vi "Drive Angle_Straight.vi"(1 "Z axis in":dbl, 2 "XAxisIn":dbl, 3 "y input":dbl) -> (8 "Z out":dbl, 9 "X0AxisOut":dbl format="%.2f", 10 "y Output":dbl)   [LabVIEW 2016]
uses:
  Robot Global Data.vi
  <vilib>/addons/control/pid/pid.llb/PID (DBL).vi
  <vilib>/addons/control/pid/pid.llb/PID Control Input Filter (DBL).vi
  <vilib>/addons/control/pid/NI_PID_pid.lvlib
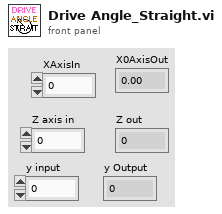
[diagram p1: front panel]
types:
  T1 = typedef "WPI_DriverStationRobotMode2.ctl" = enum16{"Autonomous Disabled", "Autonomous Enabled", "Teleop Disabled", "Teleop Enabled", "Disconnected", "Finish", "Test Disabled", "Test Enabled", "Emergency Stopped"}
  T2 = cluster{"proportional gain (Kc)":dbl, "integral time (Ti, min)":dbl, "derivative time (Td, min)":dbl}
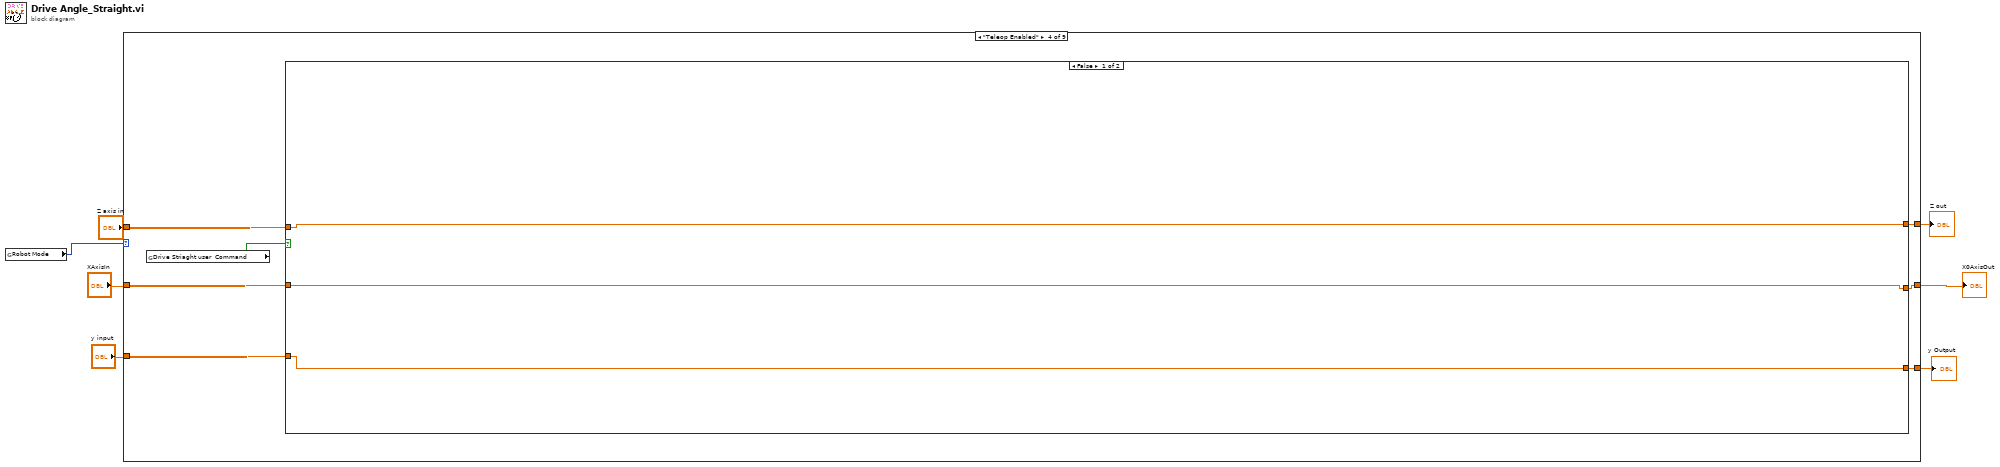
[diagram p0: block diagram]
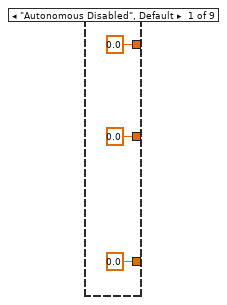
[diagram p2: hidden frame]
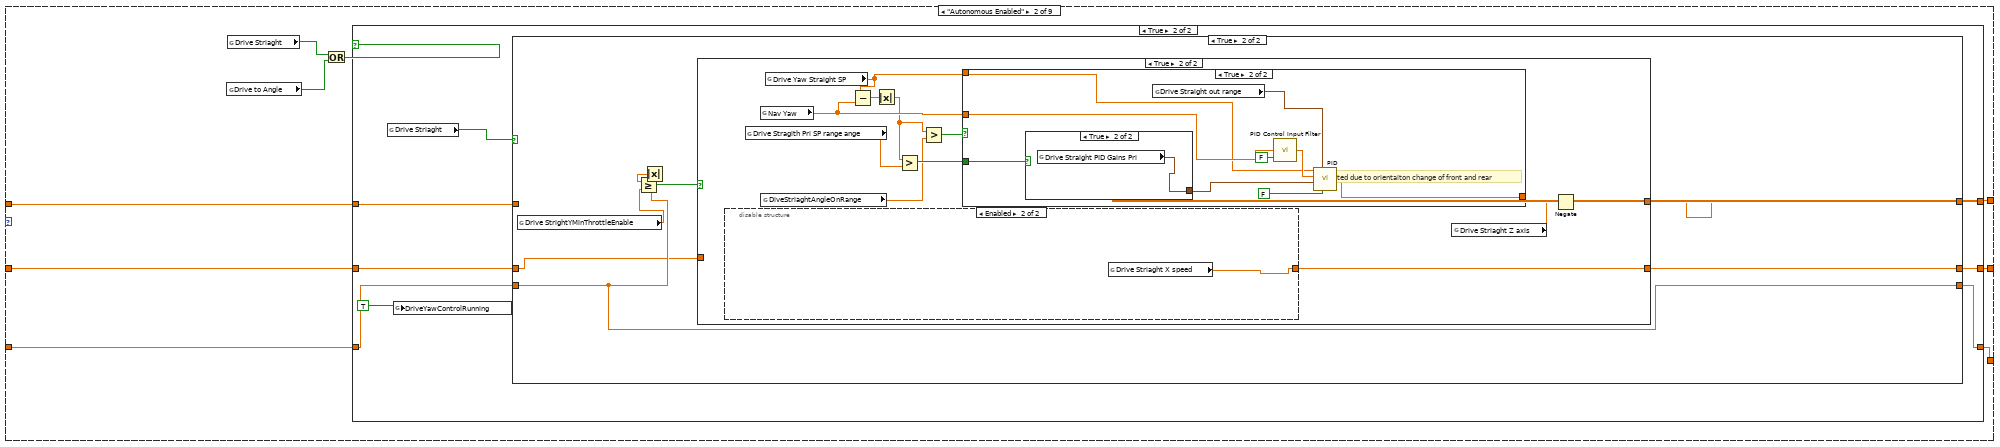
[diagram p3: hidden frame]
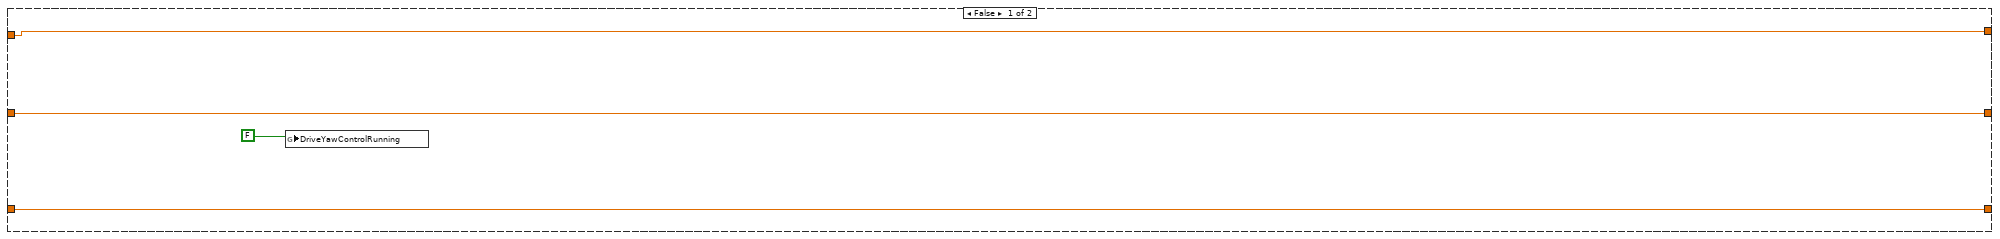
[diagram p4: hidden frame]
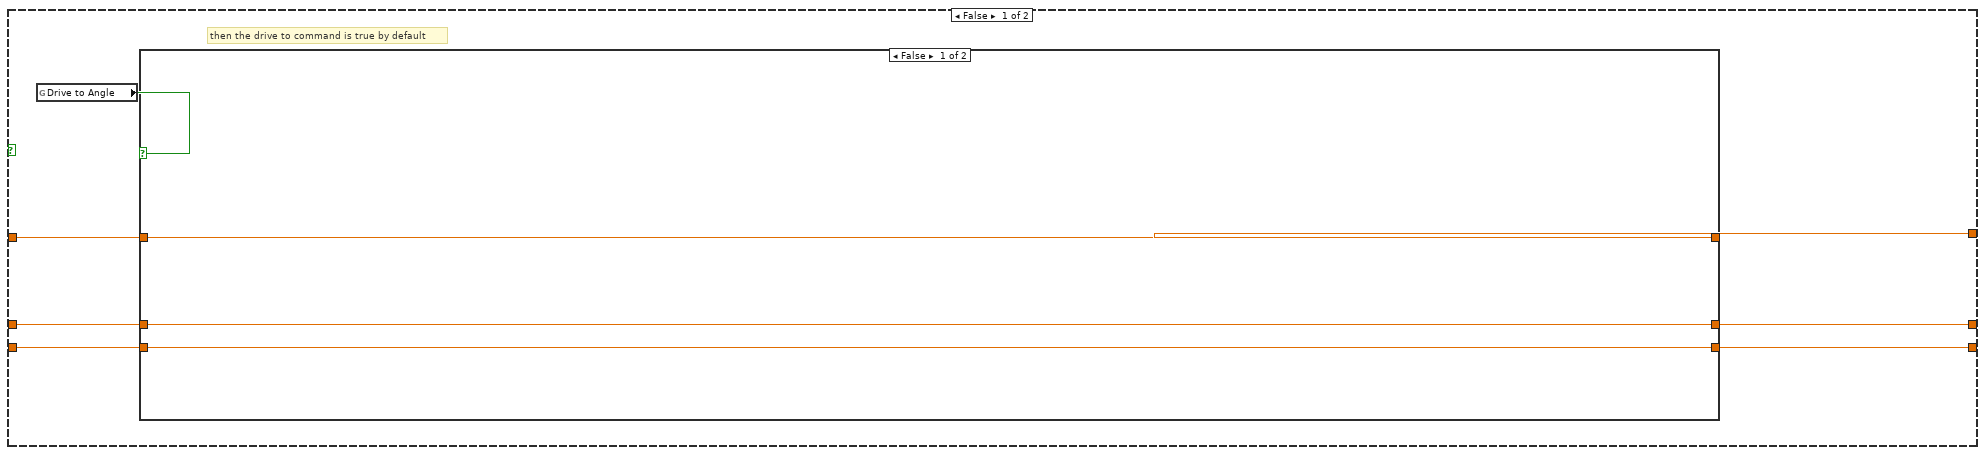
[diagram p5: hidden frame]
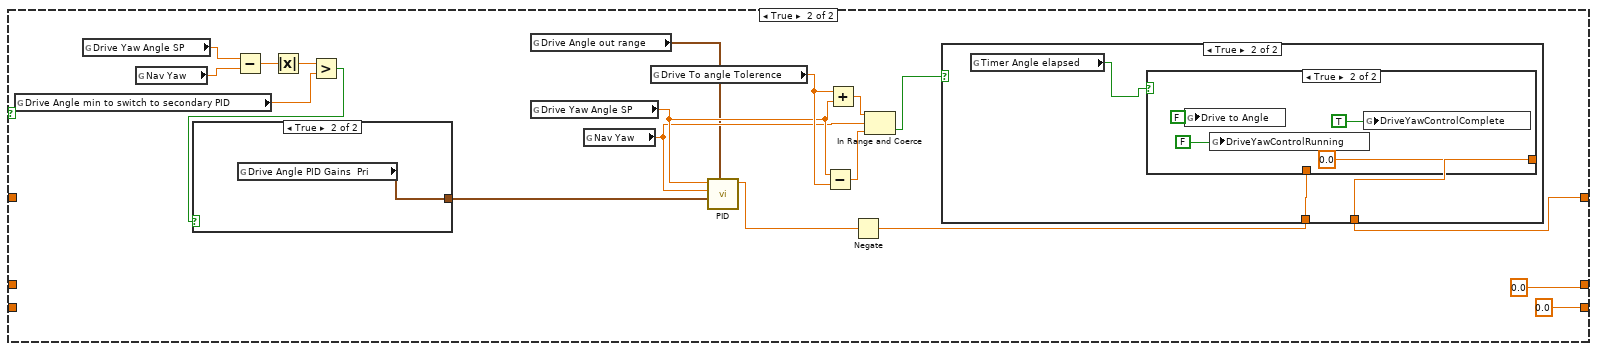
[diagram p6: hidden frame]
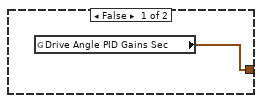
[diagram p7: hidden frame]
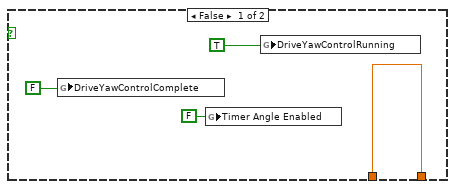
[diagram p8: hidden frame]
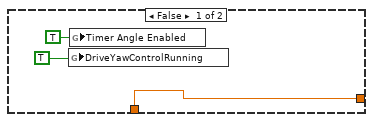
[diagram p9: hidden frame]
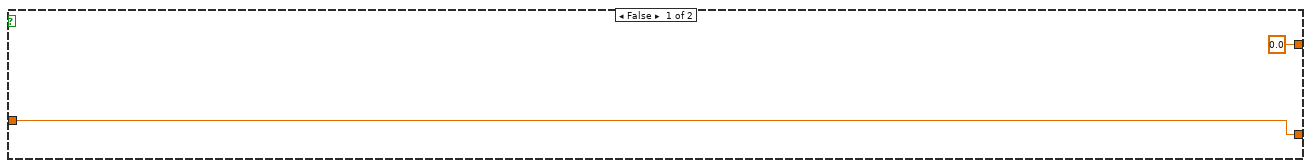
[diagram p10: hidden frame]
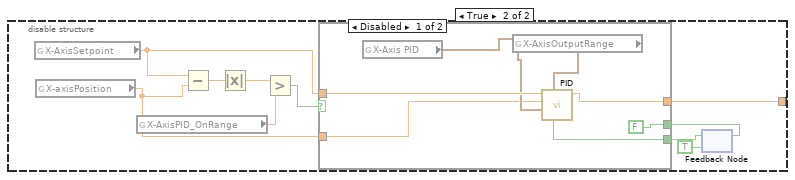
[diagram p11: hidden frame]
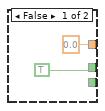
[diagram p12: hidden frame]
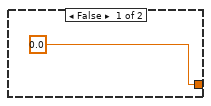
[diagram p13: hidden frame]
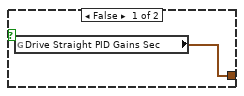
[diagram p14: hidden frame]
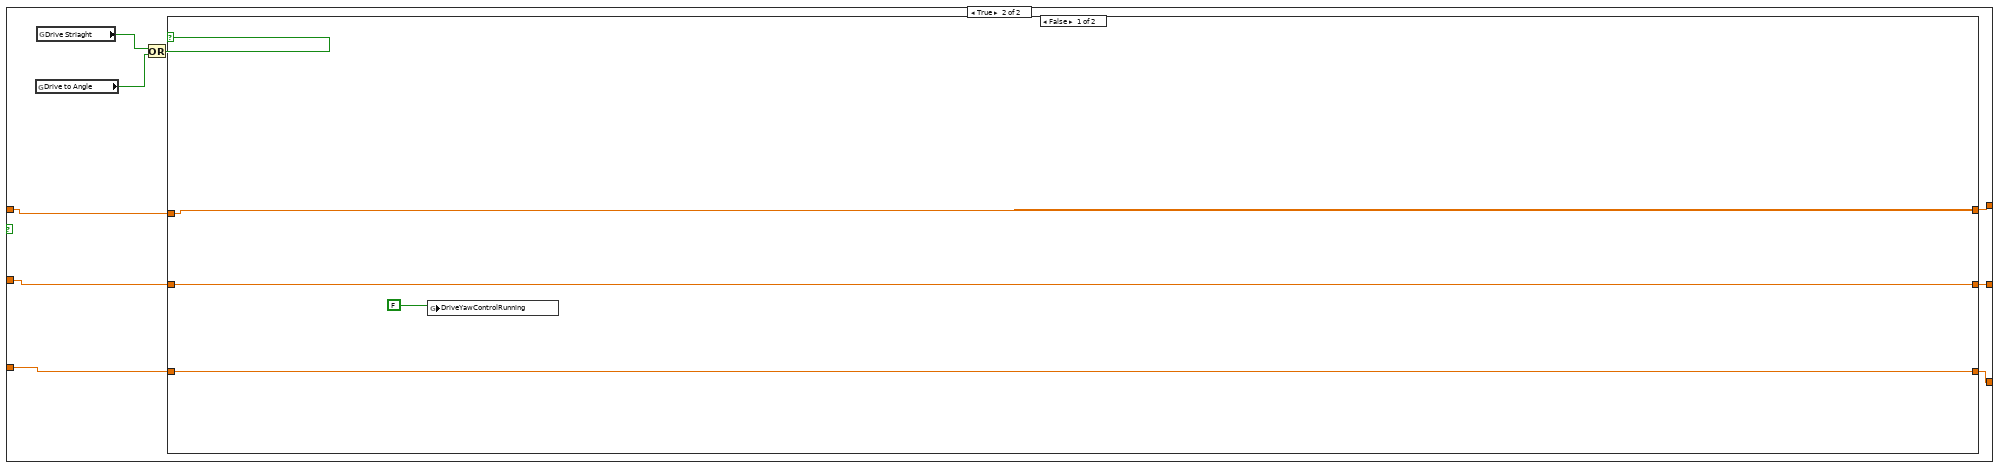
[diagram p16: hidden frame]
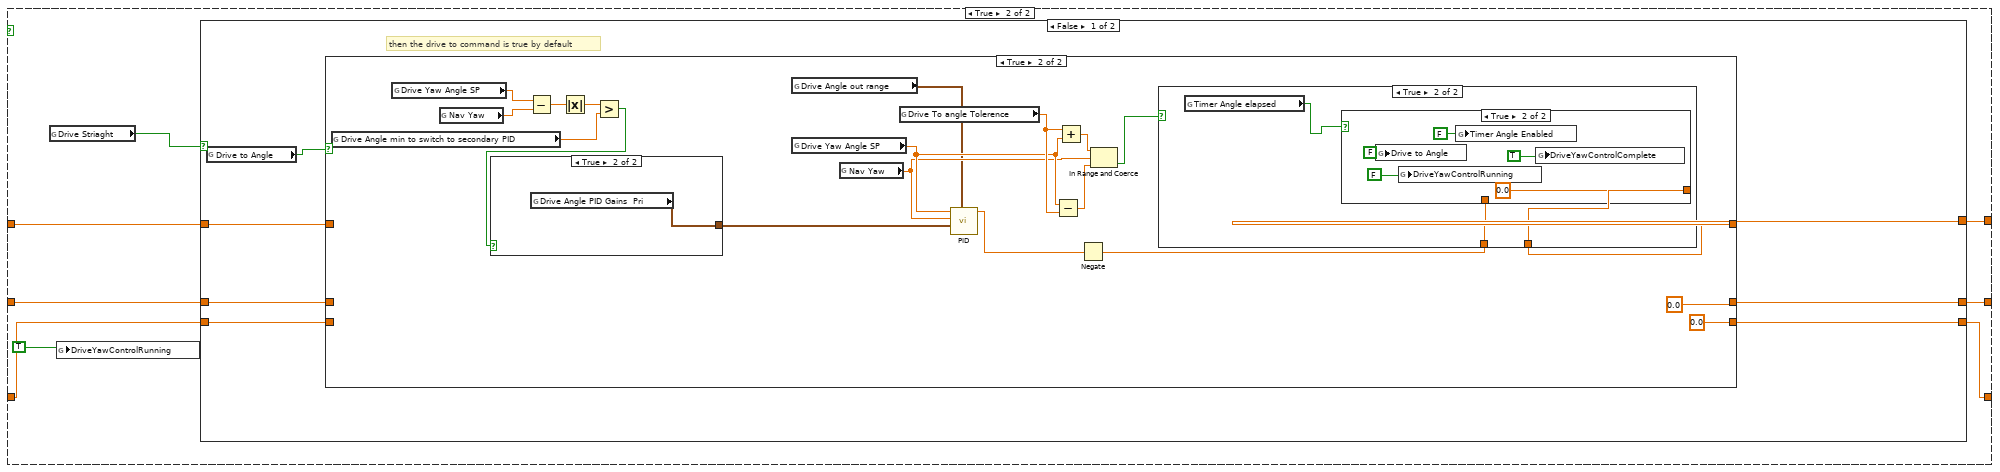
[diagram p17: hidden frame]
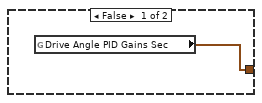
[diagram p19: hidden frame]
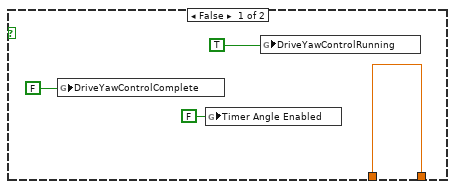
[diagram p20: hidden frame]
diagram:
  n1 = global read "Robot Global Data.vi" "Robot Mode"() -> (w1:T1)
  n2 = case shown="\"Teleop Enabled\"" w1 {
    tunnel: "Z axis in" -> [_ w19 _ w130 _ _ _ _ _]
    tunnel: [0.0 ("Z axis in") w18 _ w135 _ _ _ _ _] -> w6
    tunnel: [0.0 ("Drive Striaght X speed") w14 _ w134 _ _ _ _ _] -> w5
    tunnel: "XAxisIn" -> [_ w13 _ w131 _ _ _ _ _]
    tunnel: "y input" -> [_ w12 _ w132 _ _ _ _ _]
    tunnel: [0.0 ("y input") w11 _ w133 _ _ _ _ _] -> w2
    frame "Autonomous Disabled", Default {
    }
    frame "Autonomous Enabled" {
      n3 = global read "Robot Global Data.vi" "Drive to Angle"() -> (w17:bool)
      n4 = global read "Robot Global Data.vi" "Drive Striaght"() -> (w16:bool)
      n5 = Or(x=w16, y=w17) -> (x .or. y?=w15:bool)
      n6 = case shown="True" w15 {
        tunnel: w19 -> [w23 w29]
        tunnel: [w23 w31] -> w18
        tunnel: [w21 w27] -> w14
        tunnel: w13 -> [w21 w25]
        tunnel: [w20 w26] -> w11
        tunnel: w12 -> [w20 w24]
        frame False {
          n7 = global write "Robot Global Data.vi" "DriveYawControlRunning"(FALSE ("DriveYawControlRunning")) -> ()
        }
        frame True {
          n8 = global read "Robot Global Data.vi" "Drive Striaght"() -> (w30:bool)
          n9 = global write "Robot Global Data.vi" "DriveYawControlRunning"(TRUE ("DriveYawControlRunning")) -> ()
          n10 = case shown="True" w30 {
            tunnel: [w36 w83] -> w31
            tunnel: w29 -> [w37 _]
            tunnel: [w35 w82] -> w27
            tunnel: [w34 w80] -> w26
            tunnel: w25 -> [w33 w77]
            tunnel: w24 -> [w32 w80]
            frame False {
              # "then the drive to command is true by default"
              n11 = global read "Robot Global Data.vi" "Drive to Angle"() -> (w38:bool)
              n12 = case shown="False" w38 {
                tunnel: [w41 w54] -> w36
                tunnel: w37 -> [w41 _]
                tunnel: [w40 0.0 ("output")] -> w35
                tunnel: [w39 0.0 ("output")] -> w34
                tunnel: w33 -> [w40 _]
                tunnel: w32 -> [w39 _]
                frame False {
                }
                frame True {
                  n13 = global read "Robot Global Data.vi" "Drive Angle min to switch to secondary PID"() -> (w46:dbl)
                  n14 = global read "Robot Global Data.vi" "Drive Yaw Angle SP"() -> (w51:dbl)
                  n15 = global read "Robot Global Data.vi" "Nav Yaw"() -> (w50:dbl)
                  n16 = Subtract(x=w51, y=w50) -> (x-y=w49:dbl)
                  n17 = Absolute Value(x=w49) -> (abs(x)=w48:dbl)
                  n18 = Greater?(x=w48, y=w46) -> (0:w47:bool)
                  n19 = case shown="True" w47 {
                    tunnel: [w61 w62] -> w45
                    frame False {
                      n20 = global read "Robot Global Data.vi" "Drive Angle PID Gains Sec"() -> (w61:T2)
                    }
                    frame True {
                      n21 = global read "Robot Global Data.vi" "Drive Angle PID Gains  Pri"() -> (w62:T2)
                    }
                  }
                  n22 = global read "Robot Global Data.vi" "Drive Angle out range"() -> (w52:cluster{"output high":dbl, "output low":dbl})
                  n23 = global read "Robot Global Data.vi" "Drive Yaw Angle SP"() -> (w56:dbl)
                  n24 = global read "Robot Global Data.vi" "Nav Yaw"() -> (w53:dbl)
                  n25 = global read "Robot Global Data.vi" "Drive To angle Tolerence"() -> (w57:dbl)
                  n26 = call-poly <vilib>:"PID.vi"("output range"=w52, "PID gains"=w45, "process variable"=w53, "setpoint"=w56) -> ("output"=w60:dbl)  [unwired: 6 in, 1 out]
                  n27 = Subtract(x=w56, y=w57) -> (x-y=w58:dbl)
                  n28 = Add(x=w57, y=w56) -> (x+y=w59:dbl)
                  n29 = Negate(x=w60) -> (-x=w44:dbl)
                  n30 = In Range and Coerce(upper limit=w59, x=w53, lower limit=w58) -> (In Range?=w55:bool)  [unwired: 1 out]
                  n31 = case shown="True" w55 {
                    tunnel: w44 -> [w65 w68]
                    tunnel: [w65 w69] -> w54
                    frame False {
                      n32 = global write "Robot Global Data.vi" "DriveYawControlComplete"(FALSE ("DriveYawControlRunning")) -> ()
                      n33 = global write "Robot Global Data.vi" "Timer Angle Enabled"(FALSE ("Timer Angle Enabled")) -> ()
                      n34 = global write "Robot Global Data.vi" "DriveYawControlRunning"(TRUE ("DriveYawControlRunning")) -> ()
                    }
                    frame True {
                      n35 = global read "Robot Global Data.vi" "Timer Angle elapsed"() -> (w67:bool)
                      n36 = case shown="True" w67 {
                        tunnel: [w72 0.0] -> w69
                        tunnel: w68 -> [w72 _]
                        frame False {
                          n37 = global write "Robot Global Data.vi" "DriveYawControlRunning"(TRUE ("DriveYawControlRunning")) -> ()
                          n38 = global write "Robot Global Data.vi" "Timer Angle Enabled"(TRUE ("Timer Angle Enabled")) -> ()
                        }
                        frame True {
                          n39 = global write "Robot Global Data.vi" "Drive to Angle"(FALSE ("Drive to Angle")) -> ()
                          n40 = global write "Robot Global Data.vi" "DriveYawControlRunning"(FALSE ("DriveYawControlRunning")) -> ()
                          n41 = global write "Robot Global Data.vi" "DriveYawControlComplete"(TRUE ("DriveYawControlRunning")) -> ()
                        }
                      }
                    }
                  }
                }
              }
            }
            frame True {
              n42 = global read "Robot Global Data.vi" "Drive StrightYMinThrottleEnable"() -> (w81:dbl)
              n43 = Absolute Value(x=w80) -> (abs(x)=w78:dbl)
              n44 = Greater Or Equal?(x=w78, y=w81) -> (x >= y?=w79:bool)
              n45 = case shown="True" w79 {
                tunnel: [0.0 w87] -> w83
                tunnel: [w84 w96] -> w82
                tunnel: w77 -> [w84 _]
                frame False {
                }
                frame True {
                  n46 = disable-structure shown="Enabled" {
                    disable-tunnel: [w106 w116] -> w96
                    frame Disabled {
                      n47 = global read "Robot Global Data.vi" "X-AxisSetpoint"() -> (w105:dbl)
                      n48 = global read "Robot Global Data.vi" "X-axisPosition"() -> (w104:dbl)
                      n49 = global read "Robot Global Data.vi" "X-AxisPID_OnRange"() -> (w101:dbl)
                      n50 = Subtract(x=w105, y=w104) -> (x-y=w103:dbl)
                      n51 = Absolute Value(x=w103) -> (abs(x)=w102:dbl)
                      n52 = Greater?(x=w102, y=w101) -> (0:w100:bool)
                      n53 = feedback #1(TRUE ("reinitialize? (F)")) -> (w98:bool)
                      n54 = case shown="True" w100 {
                        tunnel: w105 -> [_ w115]
                        tunnel: [0.0 ("output") w112] -> w106
                        tunnel: w104 -> [_ w111]
                        tunnel: [TRUE FALSE ("reinitialize? (F)")] -> w99
                        tunnel: w98 -> [_ w109]
                        frame False {
                        }
                        frame True {
                          n55 = global read "Robot Global Data.vi" "X-Axis PID"() -> (w114:T2)
                          n56 = global read "Robot Global Data.vi" "X-AxisOutputRange"() -> (w113:cluster{"output high":dbl, "output low":dbl})
                          n57 = call-poly <vilib>:"PID.vi"("reinitialize? (F)"=w109, "output range"=w113, "PID gains"=w114, "process variable"=w111, "setpoint"=w115) -> ("output"=w112:dbl)  [unwired: 5 in, 1 out]
                        }
                      }
                      n58 = feedback-in #1(w99) -> ()
                    }
                    frame Enabled {
                      n59 = global read "Robot Global Data.vi" "Drive Striaght X speed"() -> (w116:dbl)
                    }
                  }
                  n60 = global read "Robot Global Data.vi" "Drive Stragith Pri SP range ange"() -> (w91:dbl)
                  n61 = global read "Robot Global Data.vi" "Nav Yaw"() -> (w95:dbl)
                  n62 = global read "Robot Global Data.vi" "DiveStriaghtAngleOnRange"() -> (w89:dbl)
                  n63 = global read "Robot Global Data.vi" "Drive Yaw Straight SP"() -> (w93:dbl)
                  n64 = Subtract(x=w93, y=w95) -> (x-y=w94:dbl)
                  n65 = Absolute Value(x=w94) -> (abs(x)=w90:dbl)
                  n66 = Greater?(x=w90, y=w91) -> (0:w92:bool)
                  n67 = Greater?(x=w90, y=w89) -> (0:w88:bool)
                  n68 = case shown="True" w88 {
                    tunnel: [0.0 ("output") w123] -> _
                    tunnel: w95 -> [_ w122]
                    tunnel: w93 -> [_ w121]
                    tunnel: w92 -> [_ w120]
                    frame False {
                    }
                    frame True {
                      # "inverted due to orientaiton change of front and rear"
                      n69 = case shown="True" w120 {
                        tunnel: [w127 w128] -> w124
                        frame False {
                          n70 = global read "Robot Global Data.vi" "Drive Straight PID Gains Sec"() -> (w127:T2)
                        }
                        frame True {
                          n71 = global read "Robot Global Data.vi" "Drive Straight PID Gains Pri"() -> (w128:T2)
                        }
                      }
                      n72 = global read "Robot Global Data.vi" "Drive Straight out range"() -> (w126:cluster{"output high":dbl, "output low":dbl})
                      n73 = call-poly <vilib>:"PID Control Input Filter.vi"("reinitialize? (F)"=FALSE, "input"=w122) -> ("output"=w125:dbl)  [unwired: 3 in]
                      n74 = call-poly <vilib>:"PID.vi"("reinitialize? (F)"=FALSE, "output range"=w126, "PID gains"=w124, "process variable"=w125, "setpoint"=w121) -> ("output"=w123:dbl)  [unwired: 5 in, 1 out]
                    }
                  }
                  n75 = global read "Robot Global Data.vi" "Drive Striaght Z axis"() -> (w86:dbl)
                  n76 = Negate(x=w86) -> (-x=w87:dbl)
                }
              }
            }
          }
        }
      }
    }
    frame "Teleop Disabled" {
    }
    frame "Teleop Enabled" {
      n77 = global read "Robot Global Data.vi" "Drive Striaght user  Command"() -> (w129:bool)
      n78 = case shown="False" w129 {
        tunnel: [w138 w144] -> w135
        tunnel: [w137 w143] -> w134
        tunnel: [w136 w142] -> w133
        tunnel: w132 -> [w136 w141]
        tunnel: w131 -> [w137 w140]
        tunnel: w130 -> [w138 w139]
        frame False {
        }
        frame True {
          n79 = global read "Robot Global Data.vi" "Drive to Angle"() -> (w147:bool)
          n80 = global read "Robot Global Data.vi" "Drive Striaght"() -> (w146:bool)
          n81 = Or(x=w146, y=w147) -> (x .or. y?=w145:bool)
          n82 = case shown="False" w145 {
            tunnel: w139 -> [w151 w157]
            tunnel: [w151 w159] -> w144
            tunnel: [w149 w155] -> w143
            tunnel: w140 -> [w149 w153]
            tunnel: [w148 w154] -> w142
            tunnel: w141 -> [w148 w152]
            frame False {
              n83 = global write "Robot Global Data.vi" "DriveYawControlRunning"(FALSE ("DriveYawControlRunning")) -> ()
            }
            frame True {
              n84 = global read "Robot Global Data.vi" "Drive Striaght"() -> (w158:bool)
              n85 = global write "Robot Global Data.vi" "DriveYawControlRunning"(TRUE ("DriveYawControlRunning")) -> ()
              n86 = case shown="False" w158 {
                tunnel: [w164 w212] -> w159
                tunnel: w157 -> [w165 _]
                tunnel: [w163 w211] -> w155
                tunnel: [w162 w209] -> w154
                tunnel: w153 -> [w161 w206]
                tunnel: w152 -> [w160 w209]
                frame False {
                  # "then the drive to command is true by default"
                  n87 = global read "Robot Global Data.vi" "Drive to Angle"() -> (w166:bool)
                  n88 = case shown="True" w166 {
                    tunnel: [w169 w182] -> w164
                    tunnel: w165 -> [w169 _]
                    tunnel: [w168 0.0 ("output")] -> w163
                    tunnel: [w167 0.0 ("output")] -> w162
                    tunnel: w161 -> [w168 _]
                    tunnel: w160 -> [w167 _]
                    frame False {
                    }
                    frame True {
                      n89 = global read "Robot Global Data.vi" "Drive Angle min to switch to secondary PID"() -> (w174:dbl)
                      n90 = global read "Robot Global Data.vi" "Drive Yaw Angle SP"() -> (w179:dbl)
                      n91 = global read "Robot Global Data.vi" "Nav Yaw"() -> (w178:dbl)
                      n92 = Subtract(x=w179, y=w178) -> (x-y=w177:dbl)
                      n93 = Absolute Value(x=w177) -> (abs(x)=w176:dbl)
                      n94 = Greater?(x=w176, y=w174) -> (0:w175:bool)
                      n95 = case shown="True" w175 {
                        tunnel: [w189 w190] -> w173
                        frame False {
                          n96 = global read "Robot Global Data.vi" "Drive Angle PID Gains Sec"() -> (w189:T2)
                        }
                        frame True {
                          n97 = global read "Robot Global Data.vi" "Drive Angle PID Gains  Pri"() -> (w190:T2)
                        }
                      }
                      n98 = global read "Robot Global Data.vi" "Drive Angle out range"() -> (w180:cluster{"output high":dbl, "output low":dbl})
                      n99 = global read "Robot Global Data.vi" "Drive Yaw Angle SP"() -> (w184:dbl)
                      n100 = global read "Robot Global Data.vi" "Nav Yaw"() -> (w181:dbl)
                      n101 = global read "Robot Global Data.vi" "Drive To angle Tolerence"() -> (w185:dbl)
                      n102 = call-poly <vilib>:"PID.vi"("output range"=w180, "PID gains"=w173, "process variable"=w181, "setpoint"=w184) -> ("output"=w188:dbl)  [unwired: 6 in, 1 out]
                      n103 = Subtract(x=w184, y=w185) -> (x-y=w186:dbl)
                      n104 = Add(x=w185, y=w184) -> (x+y=w187:dbl)
                      n105 = Negate(x=w188) -> (-x=w172:dbl)
                      n106 = In Range and Coerce(upper limit=w187, x=w181, lower limit=w186) -> (In Range?=w183:bool)  [unwired: 1 out]
                      n107 = case shown="True" w183 {
                        tunnel: w172 -> [w193 w196]
                        tunnel: [w193 w197] -> w182
                        frame False {
                          n108 = global write "Robot Global Data.vi" "DriveYawControlComplete"(FALSE ("DriveYawControlRunning")) -> ()
                          n109 = global write "Robot Global Data.vi" "Timer Angle Enabled"(FALSE ("Timer Angle Enabled")) -> ()
                          n110 = global write "Robot Global Data.vi" "DriveYawControlRunning"(TRUE ("DriveYawControlRunning")) -> ()
                        }
                        frame True {
                          n111 = global read "Robot Global Data.vi" "Timer Angle elapsed"() -> (w195:bool)
                          n112 = case shown="True" w195 {
                            tunnel: [w200 0.0] -> w197
                            tunnel: w196 -> [w200 _]
                            frame False {
                              n113 = global write "Robot Global Data.vi" "DriveYawControlRunning"(TRUE ("DriveYawControlRunning")) -> ()
                              n114 = global write "Robot Global Data.vi" "Timer Angle Enabled"(TRUE ("Timer Angle Enabled")) -> ()
                            }
                            frame True {
                              n115 = global write "Robot Global Data.vi" "Drive to Angle"(FALSE ("Drive to Angle")) -> ()
                              n116 = global write "Robot Global Data.vi" "DriveYawControlRunning"(FALSE ("DriveYawControlRunning")) -> ()
                              n117 = global write "Robot Global Data.vi" "Timer Angle Enabled"(FALSE ("Timer Angle Enabled")) -> ()
                              n118 = global write "Robot Global Data.vi" "DriveYawControlComplete"(TRUE ("DriveYawControlRunning")) -> ()
                            }
                          }
                        }
                      }
                    }
                  }
                }
                frame True {
                  n119 = global read "Robot Global Data.vi" "Drive StrightYMinThrottleEnable"() -> (w210:dbl)
                  n120 = Absolute Value(x=w209) -> (abs(x)=w207:dbl)
                  n121 = Greater Or Equal?(x=w207, y=w210) -> (x >= y?=w208:bool)
                  n122 = case shown="False" w208 {
                    tunnel: [0.0 w215] -> w212
                    tunnel: [w213 w225] -> w211
                    tunnel: w206 -> [w213 _]
                    frame False {
                    }
                    frame True {
                      n123 = disable-structure shown="Enabled" {
                        disable-tunnel: [w235 w245] -> w225
                        frame Disabled {
                          n124 = global read "Robot Global Data.vi" "X-AxisSetpoint"() -> (w234:dbl)
                          n125 = global read "Robot Global Data.vi" "X-axisPosition"() -> (w233:dbl)
                          n126 = global read "Robot Global Data.vi" "X-AxisPID_OnRange"() -> (w230:dbl)
                          n127 = Subtract(x=w234, y=w233) -> (x-y=w232:dbl)
                          n128 = Absolute Value(x=w232) -> (abs(x)=w231:dbl)
                          n129 = Greater?(x=w231, y=w230) -> (0:w229:bool)
                          n130 = feedback #2(TRUE ("reinitialize? (F)")) -> (w227:bool)
                          n131 = case shown="True" w229 {
                            tunnel: w234 -> [_ w244]
                            tunnel: [0.0 ("output") w241] -> w235
                            tunnel: w233 -> [_ w240]
                            tunnel: [TRUE FALSE ("reinitialize? (F)")] -> w228
                            tunnel: w227 -> [_ w238]
                            frame False {
                            }
                            frame True {
                              n132 = global read "Robot Global Data.vi" "X-Axis PID"() -> (w243:T2)
                              n133 = global read "Robot Global Data.vi" "X-AxisOutputRange"() -> (w242:cluster{"output high":dbl, "output low":dbl})
                              n134 = call-poly <vilib>:"PID.vi"("reinitialize? (F)"=w238, "output range"=w242, "PID gains"=w243, "process variable"=w240, "setpoint"=w244) -> ("output"=w241:dbl)  [unwired: 5 in, 1 out]
                            }
                          }
                          n135 = feedback-in #2(w228) -> ()
                        }
                        frame Enabled {
                          n136 = global read "Robot Global Data.vi" "Drive Striaght X speed"() -> (w245:dbl)
                        }
                      }
                      n137 = global read "Robot Global Data.vi" "Drive Stragith Pri SP range ange"() -> (w219:dbl)
                      n138 = global read "Robot Global Data.vi" "Nav Yaw"() -> (w223:dbl)
                      n139 = global read "Robot Global Data.vi" "DiveStriaghtAngleOnRange"() -> (w217:dbl)
                      n140 = global read "Robot Global Data.vi" "Drive Yaw Straight SP"() -> (w221:dbl)
                      n141 = Subtract(x=w221, y=w223) -> (x-y=w222:dbl)
                      n142 = Absolute Value(x=w222) -> (abs(x)=w218:dbl)
                      n143 = Greater?(x=w218, y=w219) -> (0:w220:bool)
                      n144 = Greater?(x=w218, y=w217) -> (0:w216:bool)
                      n145 = case shown="False" w216 {
                        tunnel: [0.0 ("output") w252] -> w224
                        tunnel: w223 -> [_ w251]
                        tunnel: w221 -> [_ w250]
                        tunnel: w220 -> [_ w249]
                        frame False {
                        }
                        frame True {
                          # "inverted due to orientaiton change of front and rear"
                          n146 = case shown="True" w249 {
                            tunnel: [w256 w257] -> w253
                            frame False {
                              n147 = global read "Robot Global Data.vi" "Drive Straight PID Gains Sec"() -> (w256:T2)
                            }
                            frame True {
                              n148 = global read "Robot Global Data.vi" "Drive Straight PID Gains Pri"() -> (w257:T2)
                            }
                          }
                          n149 = global read "Robot Global Data.vi" "Drive Straight out range"() -> (w255:cluster{"output high":dbl, "output low":dbl})
                          n150 = call-poly <vilib>:"PID Control Input Filter.vi"("reinitialize? (F)"=FALSE, "input"=w251) -> ("output"=w254:dbl)  [unwired: 3 in]
                          n151 = call-poly <vilib>:"PID.vi"("reinitialize? (F)"=FALSE, "output range"=w255, "PID gains"=w253, "process variable"=w254, "setpoint"=w250) -> ("output"=w252:dbl)  [unwired: 5 in, 1 out]
                        }
                      }
                      n152 = Negate(x=w224) -> (-x=w215:dbl)
                    }
                  }
                }
              }
            }
          }
        }
      }
    }
    frame "Disconnected" {
    }
    frame "Finish" {
    }
    frame "Test Disabled" {
    }
    frame "Test Enabled" {
    }
    frame "Emergency Stopped" {
    }
  }
  "Z out" <- w6
  "X0AxisOut" <- w5
  "y Output" <- w2
